vi "CPU_Port.vi"(7 "oper":T1(ring), 10 "value in":u8 format="%08b") -> (2 "value out":u8 format="%08x")   [LabVIEW 2018]
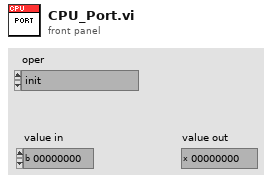
[diagram p1: front panel]
types:
  T1 = enum16{"init", "read DDR", "read PDR", "write DDR", "write PDR"}
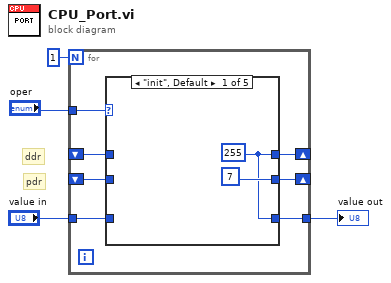
[diagram p0: block diagram]
diagram:
  # "pdr"
  # "ddr"
  n1 = for {
    N: 1 -> [_]
    shift-right: [w10] -> _
    shift-left: _ -> [w8]
    shift-right: [w9] -> _
    shift-left: _ -> [w7]
    tunnel: "oper" -> [w11]
    tunnel: [w6] -> w2
    tunnel: "value in" -> [w5]
    n2 = case shown="\"init\", Default" w11 {
      tunnel: [w12 w14 w17 w19 w21] -> w10
      tunnel: [u8 7 w15 w16 w18 w20] -> w9
      tunnel: w8 -> [_ w14 w17 _ w21]
      tunnel: w7 -> [_ w15 w16 w18 _]
      tunnel: [w12 w14 w16 w19 w20] -> w6
      tunnel: w5 -> [_ _ _ w19 w20]
      frame "init", Default {
        w12 = u8 255
      }
      frame "read DDR" {
      }
      frame "read PDR" {
      }
      frame "write DDR" {
      }
      frame "write PDR" {
      }
    }
  }
  "value out" <- w2
